vi "Configure Filter.vi"(8 "error in (no error)":errorcluster, 10 "New Filter":refnum<class "Base Filter.lvclass">, 11 "Main Display in":refnum<class "Main Display.lvclass">) -> (0 "error out":errorcluster, 3 "Main Display out":refnum<class "Main Display.lvclass">)   [LabVIEW 2016, in "Assert API Components.lvlib" / "Assert Display.lvlib" / "Main Display.lvlib" / "Main Display.lvclass"]
doc: "Creates a new filter or overwrites an existing one if a filter with the same name already exists"
uses:
  Main Display.lvclass
  Assert API Components/Filter Configurations/Base Filter.lvclass
  Assert API Components/Filter Configurations/Base Filter.lvclass/Base Filter.ctl
  Main Display.lvclass/Main Display.ctl
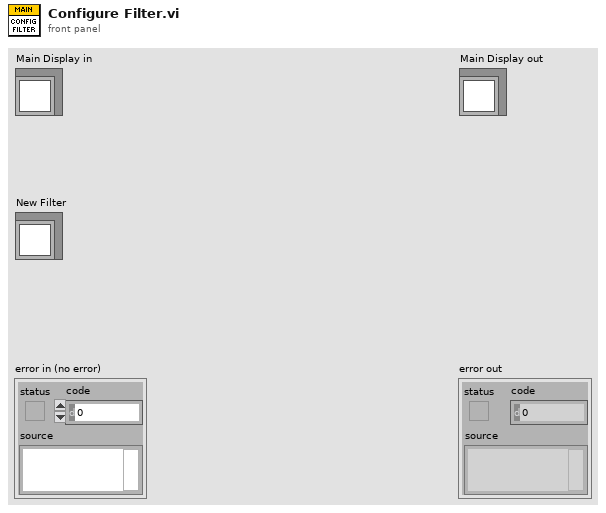
[diagram p1: front panel]
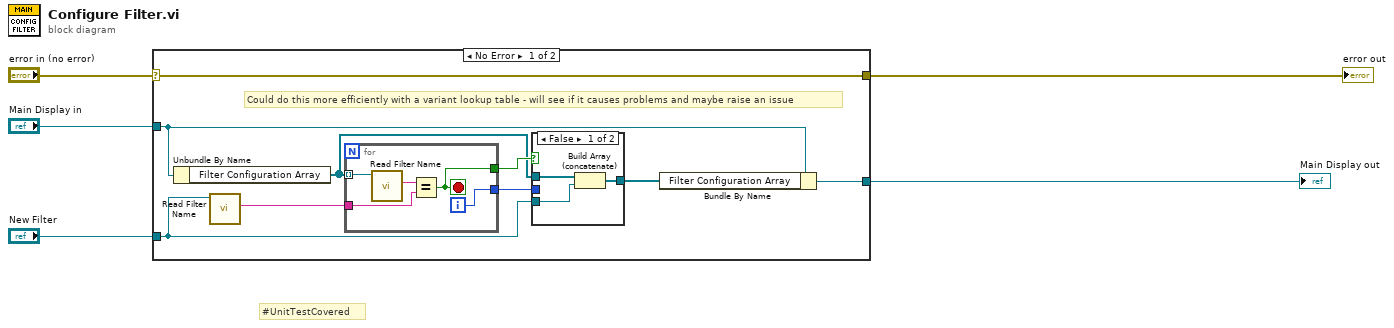
[diagram p0: block diagram]
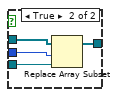
[diagram p2: hidden frame]
diagram:
  # "#UnitTestCovered"
  n1 = case shown="No Error" "error in (no error)" {
    selector: "error in (no error)" -> [w14 w28]
    tunnel: [w14 w28] -> w4
    tunnel: [w7 w27] -> w2
    tunnel: "Main Display in" -> [w13 w27]
    tunnel: "New Filter" -> [w8 _]
    frame No Error {
      # "Could do this more efficiently with a variant lookup table - will see if it causes problems and maybe raise an issue"
      n2 = Unbundle By Name(w13) -> ("Filter Configuration Array"=w10:refnum<class "Base Filter.lvclass">[])
      n3 = call "Read Filter Name.vi"("Base Filter in"=w8) -> ("Filter Name"=w12:string)  [unwired: 10 in]
      n4 = for {
        tunnel: w10 -> [w26] mode=indexing
        tunnel: w12 -> [w24]
        tunnel: [w23] -> w9
        tunnel: [w22] -> w11
        i -> [w23]
        stop <- w22 stop-if-true
        n5 = call "Read Filter Name.vi"("Base Filter in"=w26) -> ("Filter Name"=w25:string)  [unwired: 10 in]
        n6 = Equal?(x=w25, y=w24) -> (x = y?=w22:bool)
      }
      n7 = case shown="False" w11 {
        tunnel: w10 -> [w17 w21]
        tunnel: w9 -> [_ w20]
        tunnel: w8 -> [w16 w19]
        tunnel: [w15 w18] -> w6
        frame False {
          n8 = Build Array (concatenate)(w17, w16) -> (w15:refnum<class "Base Filter.lvclass">[])
        }
        frame True {
          n9 = Replace Array Subset(array=w21, new element=w19, index=w20) -> (w18:refnum<class "Base Filter.lvclass">[])
        }
      }
      n10 = Bundle By Name(cluster=w13, "Filter Configuration Array"=w6) -> (w7:refnum<class "Main Display.lvclass">)
    }
    frame Error {
    }
  }
  "error out" <- w4
  "Main Display out" <- w2
